vi "Set flags logic-at Timelapse enable event.vi"(8 "error in (no error)":errorcluster, 10 "Flag DO state":bool=TRUE) -> (0 "error out":errorcluster)   [LabVIEW 2013]
uses:
  Typedefs/Read Write Enum.ctl
  typedefs/Functions enum.ctl
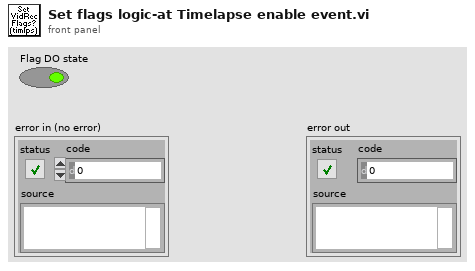
[diagram p1: front panel]
types:
  T1 = typedef "Read Write Enum.ctl" = enum16{"Read", "Write"}
  T2 = typedef "Functions enum.ctl" = enum16{"Create", "Start", "Write", "Stop", "Clear"}
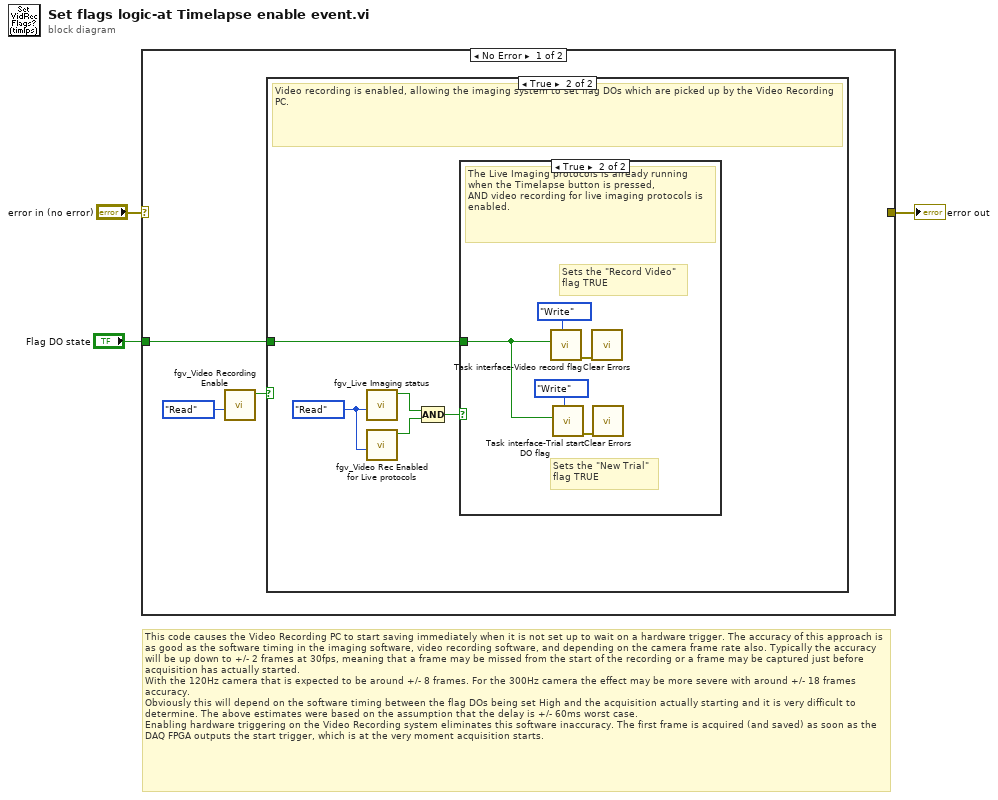
[diagram p0: block diagram]
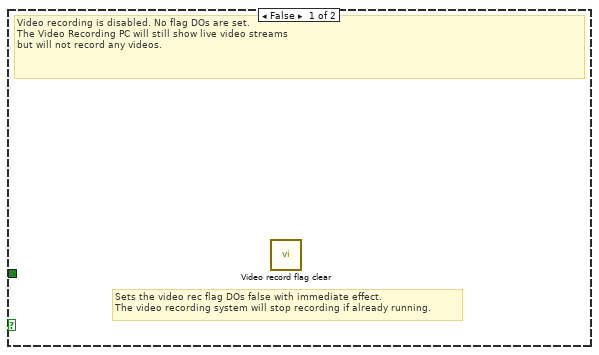
[diagram p2: hidden frame]
diagram:
  # "This code causes the Video Recording PC to start saving immediately when it is not set up to wait on a hardware trigger. The accuracy of this approach is as good as the software timing in the imaging software, video recording software, and depending on the camera frame rate also. Typically the accuracy will be up down to +/- 2 frames at 30fps, meaning that a frame may be missed from the start of the recording or a frame may be captured just before acquisition has actually started.\nWith the 120Hz camera that is expected to be around +/- 8 frames. For the 300Hz camera the effect may be more severe with around +/- 18 frames accuracy.\nObviously this will depend on the software timing between the flag DOs being set High and the acquisition actually starting and it is very difficult to determine. The above estimates were based on the assumption that the delay is +/- 60ms worst case.\nEnabling hardware triggering on the Video Recording system eliminates this software inaccuracy. The first frame is acquired (and saved) as soon as the DAQ FPGA outputs the start trigger, which is at the very moment acquisition starts."
  n1 = case shown="No Error" "error in (no error)" {
    selector: "error in (no error)" -> [_ w17]
    tunnel: [_ w17] -> w2
    tunnel: "Flag DO state" -> [w4 _]
    frame No Error {
      n2 = call "fgv_Video Recording Enable.vi"("Function"=Read_Write_Enum."Read") -> ("Video Recording Enabled"=w6:bool)  [unwired: 10 in]
      n3 = case shown="True" w6 {
        tunnel: w4 -> [_ w11]
        frame False {
          # "Sets the video rec flag DOs false with immediate effect.\nThe video recording system will stop recording if already running."
          # "Video recording is disabled. No flag DOs are set.\nThe Video Recording PC will still show live video streams \nbut will not record any videos."
          n4 = call "Video record flag clear.vi"() -> ()  [unwired: 12 in]
        }
        frame True {
          w10 = Read_Write_Enum."Read" ("Function")
          # "Video recording is enabled, allowing the imaging system to set flag DOs which are picked up by the Video Recording PC."
          n5 = call "fgv_Live Imaging status.vi"("Function"=w10) -> ("Live Imaging?"=w8:bool)  [unwired: 9 in, 1 out]
          n6 = call "fgv_Video Rec Enabled for Live protocols.vi"("Function"=w10) -> ("Video Recording Enabled for Live protocols"=w9:bool)  [unwired: 10 in]
          n7 = Compound Arithmetic op=AND(w8, w9) -> (w7:bool)
          n8 = case shown="True" w7 {
            tunnel: w11 -> [_ w12]
            frame False {
              # "Live imaging is not running,\nOR video recording for live imaging protocols is disabled."
            }
            frame True {
              # "Sets the \"New Trial\"\nflag TRUE"
              # "Sets the \"Record Video\"\nflag TRUE"
              # "The Live Imaging protocols is already running when the Timelapse button is pressed,\nAND video recording for live imaging protocols is enabled."
              n9 = call "Task interface-Video record flag.vi"("Function"=Functions_enum."Write", "DO value"=w12) -> ("error out"=w15:errorcluster)  [unwired: 9 in]
              n10 = call "Task interface-Trial start DO flag.vi"("Function"=Functions_enum."Write", "DO value"=w12) -> ("error out"=w13:errorcluster)  [unwired: 9 in]
              n11 = call <vilib>:"Clear Errors.vi"("error in (no error)"=w15) -> ()  [unwired: 6 in, 1 out]
              n12 = call <vilib>:"Clear Errors.vi"("error in (no error)"=w13) -> ()  [unwired: 6 in, 1 out]
            }
          }
        }
      }
    }
    frame Error {
    }
  }
  "error out" <- w2
